vi "Write Limit Path.vi"(8 "Error In":errorcluster, 11 "Limit File Path":path) -> (0 "Error Out":errorcluster)   [LabVIEW 2019, in "Unit Test Engine Tools.lvlib"]
uses:
  Unit Test Engine Tools.lvlib
  LVUT Global 1.vi
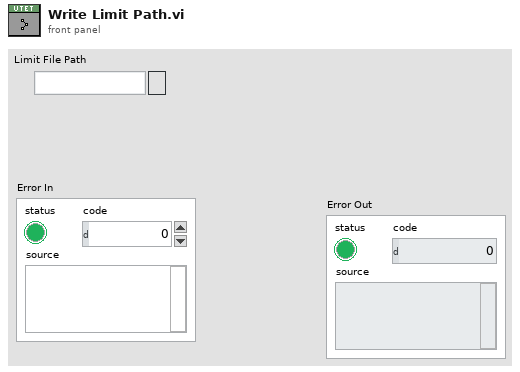
[diagram p1: front panel]
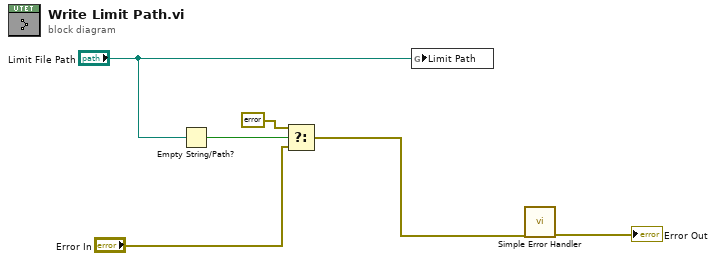
[diagram p0: block diagram]
diagram:
  n1 = Empty String/Path?(string/path="Limit File Path") -> (empty?=w5:bool)
  n2 = Select(t=errorcluster {"status"=TRUE, "code"=-1000001, "source"="Is empty path !"}, s=w5, f="Error In") -> (s? t:f=w3:errorcluster)
  n3 = global write "LVUT Global 1.vi" "Limit Path"("Limit File Path") -> ()
  n4 = call <vilib>:"Simple Error Handler.vi"("error in (no error)"=w3) -> ("error out"=→"Error Out":errorcluster)  [unwired: 4 in, 4 out]
